vi "build_command_string.vi"(11 "key state":bool[](array[boolean])) -> (3 "command":string)   [LabVIEW 2025]
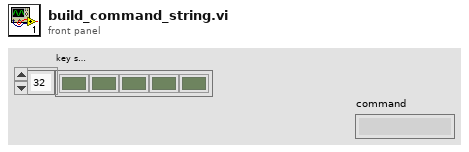
[diagram p1: front panel]
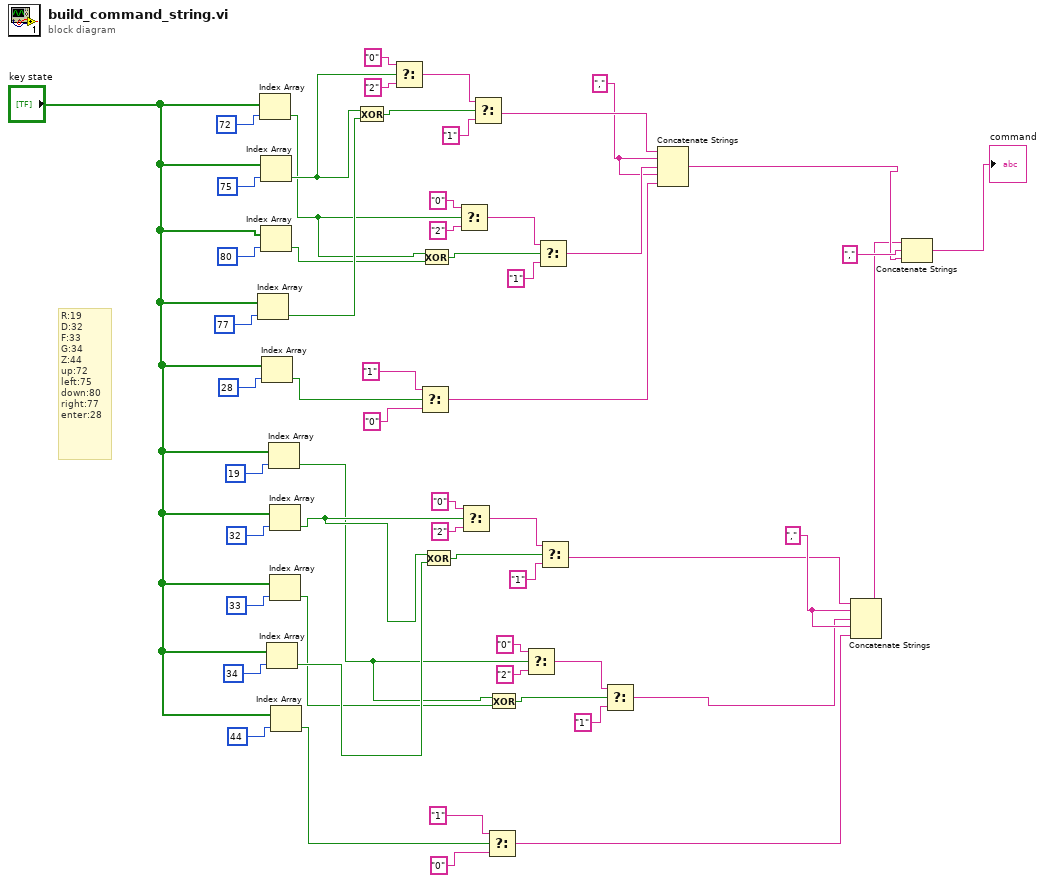
[diagram p0: block diagram]
diagram:
  w8 = ","
  w27 = ","
  # "R:19\nD:32\nF:33\nG:34\nZ:44\nup:72\nleft:75\ndown:80\nright:77\nenter:28"
  n1 = Index Array(array="key state", index=77) -> (element=w41:bool)
  n2 = Index Array(array="key state", index=72) -> (element=w31:bool)
  n3 = Index Array(array="key state", index=75) -> (element=w40:bool)
  n4 = Index Array(array="key state", index=80) -> (element=w30:bool)
  n5 = Index Array(array="key state", index=28) -> (element=w46:bool)
  n6 = Index Array(array="key state", index=34) -> (element=w12:bool)
  n7 = Index Array(array="key state", index=19) -> (element=w9:bool)
  n8 = Index Array(array="key state", index=32) -> (element=w11:bool)
  n9 = Index Array(array="key state", index=33) -> (element=w10:bool)
  n10 = Index Array(array="key state", index=44) -> (element=w13:bool)
  n11 = Exclusive Or(1:w41, 2:w40) -> (0:w43:bool)
  n12 = Select(t="0", s=w40, f="2") -> (s? t:f=w37:string)
  n13 = Select(t="1", s=w46, f="0") -> (s? t:f=w26:string)
  n14 = Exclusive Or(1:w30, 2:w31) -> (0:w32:bool)
  n15 = Exclusive Or(1:w12, 2:w11) -> (0:w16:bool)
  n16 = Select(t="0", s=w31, f="2") -> (s? t:f=w36:string)
  n17 = Select(t="0", s=w11, f="2") -> (s? t:f=w20:string)
  n18 = Select(t=w37, s=w43, f="1") -> (s? t:f=w29:string)
  n19 = Select(t="1", s=w13, f="0") -> (s? t:f=w5:string)
  n20 = Exclusive Or(1:w10, 2:w9) -> (0:w25:bool)
  n21 = Select(t="0", s=w9, f="2") -> (s? t:f=w21:string)
  n22 = Select(t=w36, s=w32, f="1") -> (s? t:f=w28:string)
  n23 = Select(t=w20, s=w16, f="1") -> (s? t:f=w7:string)
  n24 = Select(t=w21, s=w25, f="1") -> (s? t:f=w6:string)
  n25 = Concatenate Strings(w29, w27, w28, w27, w26) -> (w2:string)
  n26 = Concatenate Strings(w7, w8, w6, w8, w5) -> (w1:string)
  n27 = Concatenate Strings(w1, "," ("string"), w2) -> (→"command":string)
